vi "S2C_FORNAX_Proc_ManageMsgClear.vi"(7 "Msg In":T1, 8 "Error In":errorcluster) -> (0 "Error Out":errorcluster, 5 "Msg Out":T1)   [LabVIEW 2015]
doc: "Keeps the ViperMsg and DDSMsg arrays to 1000 characters or less."
uses:
  S2C_FORNAX_Proc_Globals.vi
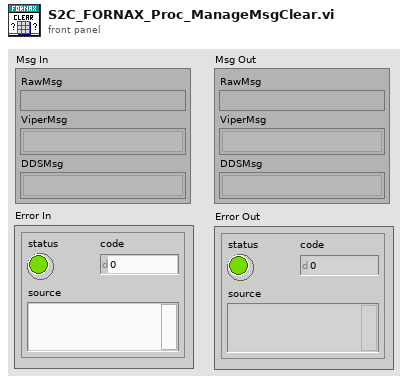
[diagram p1: front panel]
types:
  T1 = cluster{"RawMsg":string, "ViperMsg":string[], "DDSMsg":string[]}
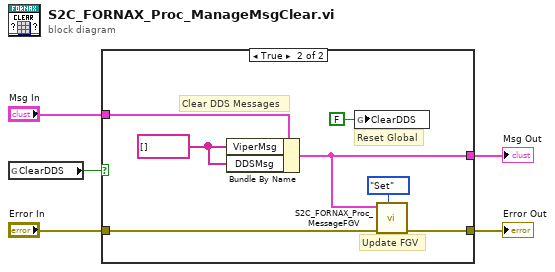
[diagram p0: block diagram]
diagram:
  n1 = global read "S2C_FORNAX_Proc_Globals.vi" "ClearDDS"() -> (w3:bool)
  n2 = case shown="True" w3 {
    tunnel: "Msg In" -> [w7 w14]
    tunnel: [w7 w8] -> w4
    tunnel: "Error In" -> [w6 w10]
    tunnel: [w6 w9] -> w1
    frame False {
    }
    frame True {
      w13 = string[] [] ("ViperMsg")
      # "Update FGV"
      # "Reset Global"
      # "Clear DDS Messages"
      n3 = Bundle By Name(cluster=w14, "ViperMsg"=w13, "DDSMsg"=w13) -> (w8:T1)
      n4 = global write "S2C_FORNAX_Proc_Globals.vi" "ClearDDS"(FALSE ("ClearDDS")) -> ()
      n5 = call "S2C_FORNAX_Proc_MessageFGV.vi"("Action"=enum16{"Set", "Get"}."Set", "Error In"=w10, "Msg In"=w8) -> ("Error Out"=w9:errorcluster)  [unwired: 7 in, 1 out]
    }
  }
  "Error Out" <- w1
  "Msg Out" <- w4
